vi "Sequence Settings Cluster to Number.vi"(1 "Settings":T1) -> (0 "Sequence Settings":i32)   [LabVIEW 2011]
uses:
  Sequence Settings.ctl
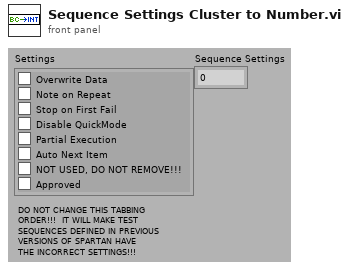
[diagram p1: front panel]
types:
  T1 = typedef "Sequence Settings.ctl" = cluster{"Overwrite Data":bool, "Note on Repeat":bool, "Stop on First Fail":bool, "Disable QuickMode":bool, "Partial Execution":bool, "Auto Next Item":bool, "NOT USED, DO NOT REMOVE!!!":bool, "Approved":bool}
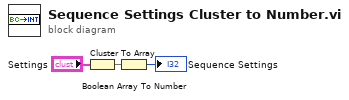
[diagram p0: block diagram]
diagram:
  n1 = Cluster To Array(cluster="Settings") -> (array=w2:bool[])
  n2 = Boolean Array To Number(Boolean array=w2) -> (number=→"Sequence Settings":u32)
